vi "densitySamp (SubVI).vi"(10 "dimention":cluster{"x dim":dbl, "y dim":dbl}={"x dim"=40.0, "y dim"=40.0}, 11 "density":i32=200) -> (3 "samples":i32)   [LabVIEW 2011]
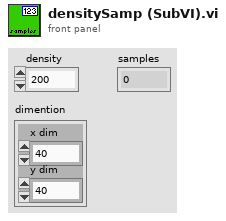
[diagram p1: front panel]
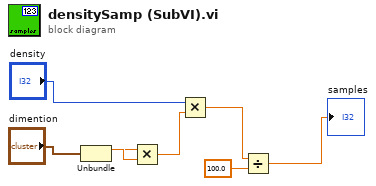
[diagram p0: block diagram]
diagram:
  n1 = Unbundle("dimention") -> ("x dim"=w7:dbl, "y dim"=w6:dbl)
  n2 = Multiply(x=w6, y=w7) -> (x*y=w5:dbl)
  n3 = Multiply(x="density", y=w5) -> (x*y=w3:dbl)
  n4 = Divide(x=w3, y=100.0) -> (x/y=→"samples":dbl)
